vi "SailAndRudderArbiter.vi"() -> ()   [LabVIEW 2012]
doc: "Eric Schneider and Bonnie Ishiguro\nJan. 2014\n\nThis arbiter takes in a number of suggestions on how to set the sails and rudder, then decides which suggestions to pay attention to at any given time. The two most common modes, most likely, are 'Straight' and 'Turning', and they are a blend of a simple sail lookup based on relative wind and various other suggestions. 'Straight' tries to blend in rudder force balancing and luff removal, and 'Turning' tries to blend in overpowering and underpowering certain sails to get the boats to turn. Those 'blend' blocks are yet to be written, so right now all suggestions except the wind-to-sail lookup are multiplied by 0.\n\nSemi-hardcoded maneuvers involving both the sails and rudder, like tacks or jibes, are also done in this arbiter. In those cases the suggestions for how to do a tack become the only command the boat pays attention to, including for the rudder. Normally the rudder is driven by a control loop around the boat heading, but in a maneuver (tack, jibe), the rudder and sails are controlled by the logic in the MidBrain Think code found in SailSetSuggestions.vi.\n\nThe expected inputs are typedefs, all constrained between 0-1. This shouldn't be changed without also altering the algorithms."
uses:
  Data/TypeDefs/Rudder Set Suggestions.ctl
  Data/TypeDefs/Sail Set Suggestions.ctl
  Data/TypeDefs/MB Think to Act Bundled Sail Commands.ctl
panel:
  out "RudderSetpoint":T1 min=-1.0 max=1.0
  out "SailSetpoints":T2 {"MainSailSuggestion" min=0.0 max=1.0; "JibSailSuggestion" min=0.0 max=1.0}
  in  "SailSuggestionToMB-ACTArbiter":T3 {"SailByWindLookup"."MainSailSuggestion" min=0.0 max=1.0; "SailByWindLookup"."JibSailSuggestion" min=0.0 max=1.0; "SailsByTurningBoat"."MainSailSuggestion" min=0.0 max=1.0; "SailsByTurningBoat"."JibSailSuggestion" min=0.0 max=1.0; "SailByTurtleMode"."MainSailSuggestion" min=0.0 max=1.0; "SailByTurtleMode"."JibSailSuggestion" min=0.0 max=1.0; "RudderByTurtleMode" min=-1.0 max=1.0; "SailsByReducingLuffing"."MainSailSuggestion" min=0.0 max=1.0; "SailsByReducingLuffing"."JibSailSuggestion" min=0.0 max=1.0; "SailsByBalancingRudder"."MainSailSuggestion" min=0.0 max=1.0; "SailsByBalancingRudder"."JibSailSuggestion" min=0.0 max=1.0; "TackManeuverSails"."MainSailSuggestion" min=0.0 max=1.0; "TackManeuverSails"."JibSailSuggestion" min=0.0 max=1.0; "TackManeuverRudder" min=-1.0 max=1.0; "JibeManeuverSails"."MainSailSuggestion" min=0.0 max=1.0; "JibeManeuverSails"."JibSailSuggestion" min=0.0 max=1.0; "JibeManeuverRudder" min=-1.0 max=1.0}
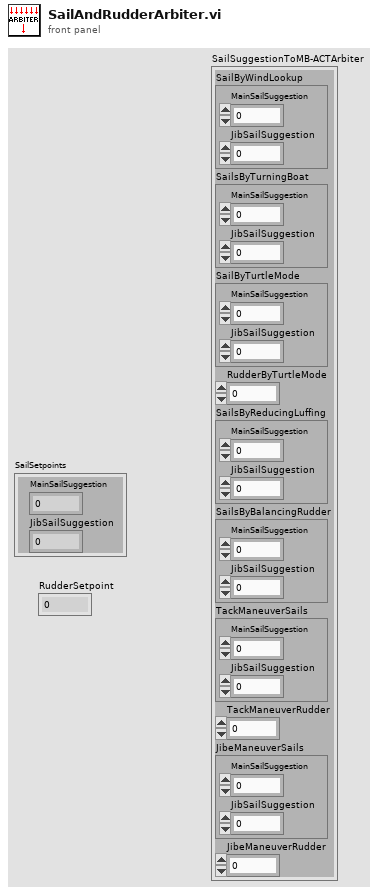
[diagram p1: front panel]
types:
  T1 = typedef "Rudder Set Suggestions.ctl" = dbl
  T2 = typedef "Sail Set Suggestions.ctl" = cluster{"MainSailSuggestion":dbl, "JibSailSuggestion":dbl}
  T3 = typedef "MB Think to Act Bundled Sail Commands.ctl" = cluster{"SailByWindLookup":T2, "SailsByTurningBoat":T2, "SailByTurtleMode":T2, "RudderByTurtleMode":T1, "SailsByReducingLuffing":T2, "SailsByBalancingRudder":T2, "TackManeuverSails":T2, "TackManeuverRudder":T1, "JibeManeuverSails":T2, "JibeManeuverRudder":T1}
  T4 = typedef "Sailing State of Boat.ctl" = enum16{"Straight", "Turning", "Approach Maneuver", "Cross Wind (Tack)", "Cross Wind (Gybe)", "Turtle Mode", ""}
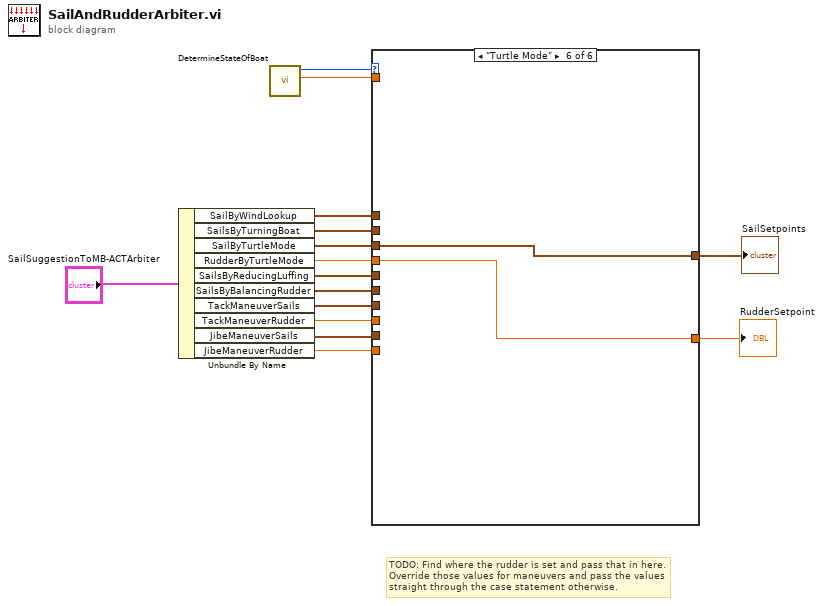
[diagram p0: block diagram]
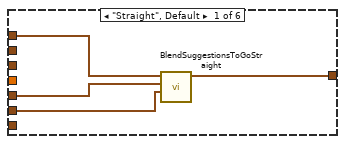
[diagram p2: hidden frame]
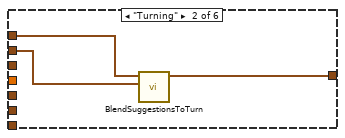
[diagram p3: hidden frame]
diagram:
  # "TODO: Find where the rudder is set and pass that in here.\nOverride those values for maneuvers and pass the values\nstraight through the case statement otherwise."
  n1 = Unbundle By Name("SailSuggestionToMB-ACTArbiter") -> ("SailByWindLookup"=w12:T2, "SailsByTurningBoat"=w8:T2, "SailByTurtleMode"=w3:T2, "RudderByTurtleMode"=w2:T1, "SailsByReducingLuffing"=w11:T2, "SailsByBalancingRudder"=w10:T2, "TackManeuverSails"=w7:T2, "TackManeuverRudder"=w6:T1, "JibeManeuverSails"=w1:T2, "JibeManeuverRudder"=w4:T1)
  n2 = call "DetermineStateOfBoat.vi"() -> ("TimeSpentInCurrentState"=w13:dbl, "StateOfBoat"=w15:T4)  [unwired: 9 in]
  n3 = case shown="\"Turtle Mode\"" w15 {
    tunnel: [w19 w20 w23 w25 w27 w29] -> w9
    tunnel: w13 -> [_ _ _ _ _ _]
    tunnel: w12 -> [w18 w22 w23 _ _ _]
    tunnel: w11 -> [w17 _ _ _ _ _]
    tunnel: w10 -> [w16 _ _ _ _ _]
    tunnel: w8 -> [_ w21 _ _ _ _]
    tunnel: w7 -> [_ _ _ w25 _ _]
    tunnel: w6 -> [_ _ _ w24 _ _]
    tunnel: [_ _ _ w24 w26 w28] -> w5
    tunnel: w1 -> [_ _ _ _ w27 _]
    tunnel: w4 -> [_ _ _ _ w26 _]
    tunnel: w3 -> [_ _ _ _ _ w29]
    tunnel: w2 -> [_ _ _ _ _ w28]
    frame "Straight", Default {
      n4 = call "BlendSuggestionsToGoStraight.vi"("BalanceRudderSailSuggestion"=w16, "LuffToSailSuggestion"=w17, "WindToSailLookup"=w18) -> ("BlendedGoStraightSailSetting"=w19:T2)  [unwired: 8 in]
    }
    frame "Turning" {
      n5 = call "BlendSuggestionsToTurn.vi"("SailsByTurningBoat"=w21, "WindToSailLookup"=w22) -> ("BlendedTurningSailSetting"=w20:T2)  [unwired: 9 in]
    }
    frame "Approach Maneuver" {
    }
    frame "Cross Wind (Tack)" {
      # "Use the tack suggestions here!"
    }
    frame "Cross Wind (Gybe)" {
      # "Use the jibe suggestions here!"
    }
    frame "Turtle Mode" {
    }
  }
  "SailSetpoints" <- w9
  "RudderSetpoint" <- w5
